vi "Update Value by Name.vi"(7 "Overwrite? (F)":bool, 8 "error in (no error)":errorcluster, 9 "Value":variant, 10 "Name":string, 11 "Processing in":refnum<class "Processing.lvclass">) -> (0 "error out":errorcluster, 3 "Processing out":refnum<class "Processing.lvclass">)   [LabVIEW 2020, in "HTTP Server.lvlib" / "Processing.lvclass"]
uses:
  Processing.lvclass
  Processing.lvclass/Processing.ctl
  Values/Values.lvclass
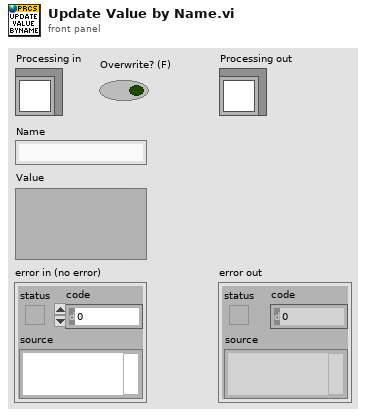
[diagram p1: front panel]
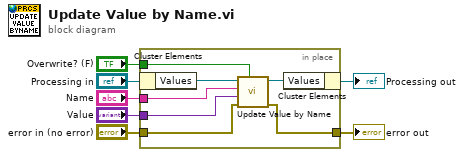
[diagram p0: block diagram]
diagram:
  n1 = in-place {
    in-place-border: "Overwrite? (F)" -> [w13]
    in-place-border: "Name" -> [w9]
    in-place-border: "error in (no error)" -> [w11]
    in-place-border: [w10] -> w3
    in-place-border: "Value" -> [w8]
    n2 = in-place-cluster #1("Processing in") -> ("Values"=w14:refnum<class "Values.lvclass">)
    n3 = call "Update Value by Name.vi"("Overwrite? (F)"=w13, "error in (no error)"=w11, "Value"=w8, "Name"=w9, "Values in"=w14) -> ("error out"=w10:errorcluster, "Values out"=w12:refnum<class "Values.lvclass">)  [unwired: 5 in]
    n4 = in-place-cluster #1("Values"=w12) -> (→"Processing out":refnum<class "Processing.lvclass">)
  }
  "error out" <- w3
